vi "Execution Profiler View.vi"(8 "error in (no error)":errorcluster, 10 "Timing Results":map{string, dbl}(c390)) -> (0 "error out":errorcluster)   [LabVIEW 2020, in "Execution Profiler.lvlib" / "Execution Profiler.lvclass"]
uses:
  Execution Profiler.lvclass
  Execution Profiler.lvclass/Execution Profiler.ctl
panel:
  in  "Method Test Times":i32(listbox)
  out "Histogram":cluster{"X":dbl, "Y":dbl}[](graph)
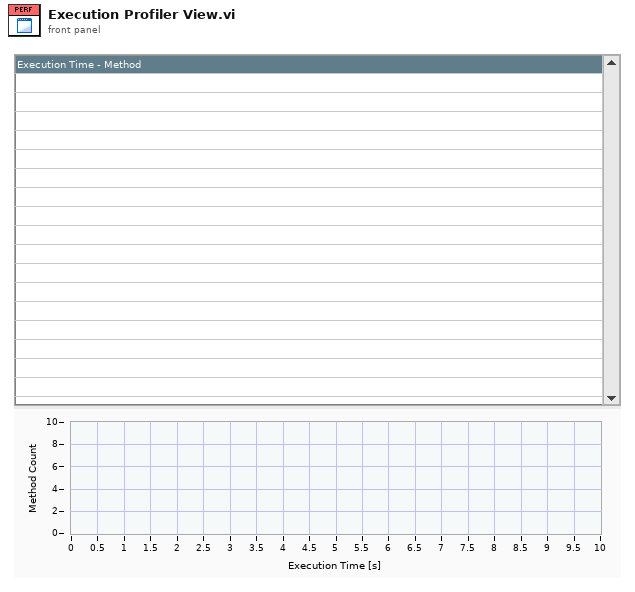
[diagram p1: front panel]
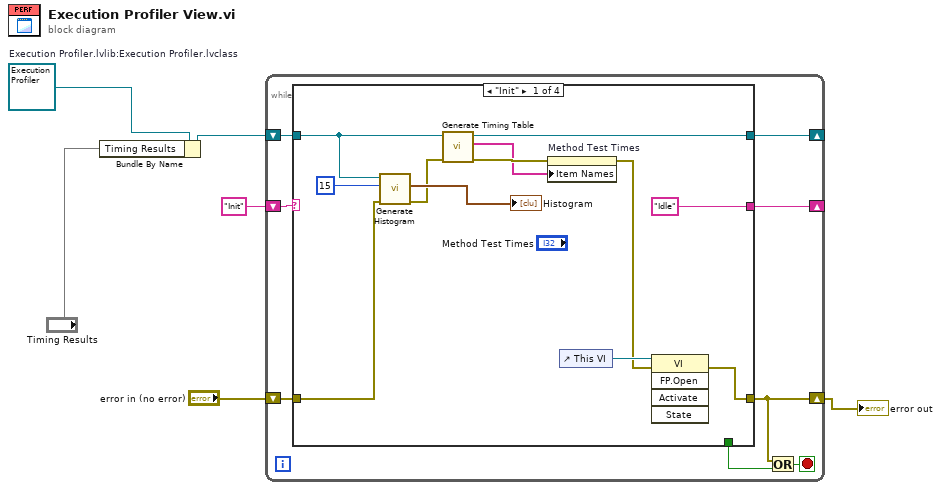
[diagram p0: block diagram]
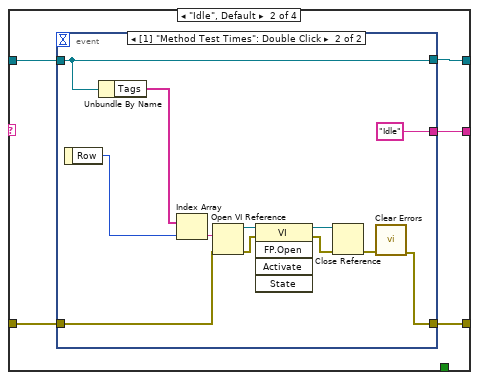
[diagram p2: hidden frame]
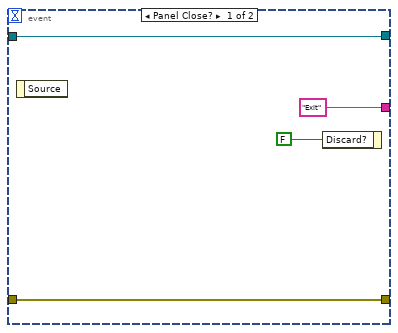
[diagram p3: hidden frame]
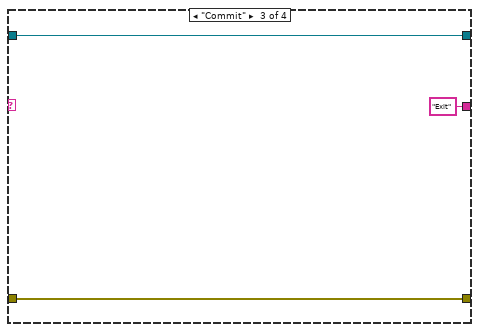
[diagram p4: hidden frame]
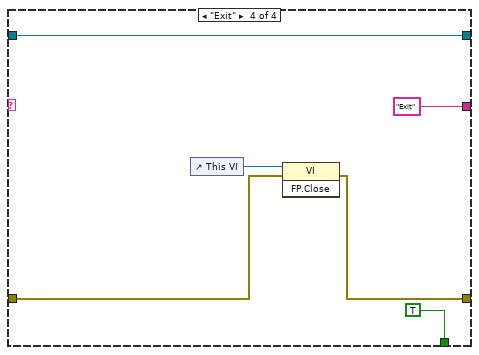
[diagram p5: hidden frame]
diagram:
  w2 = refnum<class "Execution Profiler.lvclass"> refnum  # Execution Profiler.lvlib:Execution Profiler.lvclass
  n1 = Bundle By Name(cluster=w2, "Timing Results"="Timing Results") -> (w3:refnum<class "Execution Profiler.lvclass">)
  n2 = while {
    shift-right: [w11] -> _
    shift-left: w3 -> [w12]
    shift-right: [w7] -> w4
    shift-left: "error in (no error)" -> [w13]
    shift-right: [w10] -> _
    shift-left: "Init" -> [w14]
    stop <- w8 stop-if-true
    n3 = case shown="\"Init\"" w14 {
      tunnel: [w21 w31 w50 w52] -> w7
      tunnel: w13 -> [w24 w30 w50 w51]
      tunnel: w12 -> [w15 w29 w49 w56]
      tunnel: [w20 w28 w49 w56] -> w11
      tunnel: ["Idle" w27 "Exit" "Exit"] -> w10
      tunnel: [_ _ _ TRUE] -> w9
      frame "Init" {
        n4 = call "Generate Histogram.vi"("error in (no error)"=w24, "Interval Scaling"=u8 15 ("Number of intervals"), "View In"=w15) -> ("error out"=w19:errorcluster, "Histogram"=→"Histogram":cluster{dbl, dbl}[])  [unwired: 7 in]
        n5 = call "Generate Timing Table.vi"("error in (no error)"=w19, "Performance Analyzer In"=w15) -> ("error out"=w18:errorcluster, "Timing List"=w16:string[], "Performance Analyzer Out"=w20:refnum<class "Execution Profiler.lvclass">)  [unwired: 7 in]
        n6 = property on="Method Test Times" class="LstBox (strict)"(error in=w18, "Item Names"=w16) -> (error out=w17:errorcluster)  [unwired: 1 in, 1 out]
        n7 = control-ref of="This VI"() -> (w22:refnum<vi>)
        n8 = invoke class="VI" method="FP.Open"(reference=w22, error in=w17) -> (error out=w21:errorcluster)  [unwired: 3 in, 4 out]
      }
      frame "Idle", Default {
        n9 = event shown="[1] \"Method Test Times\": Double Click" {
          selector: _ -> [_ _]
          dyn-events: _ -> [_ _]
          timeout: _ -> [_ _]
          tunnel: [w35 w36] -> w31
          tunnel: w30 -> [w35 w38]
          tunnel: w29 -> [w34 w45]
          tunnel: [w34 w45] -> w28
          tunnel: ["Exit" "Idle"] -> w27
          event Panel Close? {
            n10 = event-data() -> ()  [unwired: 1 in, 1 out]
            n11 = event-data("Discard?"=FALSE) -> ()  [unwired: 1 in, 1 out]
          }
          event "Method Test Times": Double Click {
            n12 = event-data() -> ("Row"=w46:i32)  [unwired: 1 in]
            n13 = Unbundle By Name(w45) -> ("Tags"=w44:string[])
            n14 = Index Array(array=w44, index=w46) -> (element=w43:string)
            n15 = Open VI Reference(vi path=w43, error in (no error)=w38) -> (vi reference=w42:refnum<vi>, error out=w39:errorcluster)  [unwired: 4 in]
            n16 = invoke class="VI" method="FP.Open"(reference=w42, error in=w39) -> (reference out=w41:refnum<vi>, error out=w40:errorcluster)  [unwired: 3 in, 3 out]
            n17 = Close Reference(reference=w41, error in (no error)=w40) -> (error out=w37:errorcluster)
            n18 = call <vilib>:"Clear Errors.vi"("error in (no error)"=w37) -> ("error out"=w36:errorcluster)  [unwired: 5 in, 1 out]
          }
        }
      }
      frame "Commit" {
      }
      frame "Exit" {
        n19 = control-ref of="This VI"() -> (w53:refnum<vi>)
        n20 = invoke class="VI" method="FP.Close"(reference=w53, error in=w51) -> (error out=w52:errorcluster)  [unwired: 1 in, 2 out]
      }
    }
    n21 = Or(x=w7, y=w9) -> (x .or. y?=w8:bool)
  }
  "error out" <- w4
